vi "Remove HTML Tags from String.vi"(1 "HTML text":string) -> (0 "HTML text w/o tags":string)   [LabVIEW 2021, in "Strings.lvlib"]
uses:
  Strings/Strings.lvlib
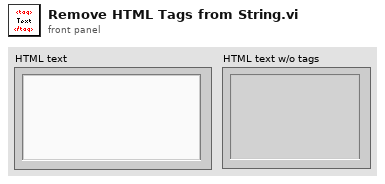
[diagram p1: front panel]
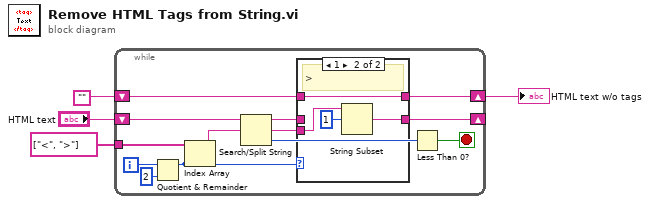
[diagram p0: block diagram]
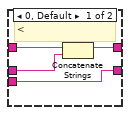
[diagram p2: hidden frame]
diagram:
  n1 = while {
    shift-right: [w7] -> _
    shift-left: "HTML text" -> [w17]
    tunnel: string[] ["<", ">"] ("search string/char (-)") -> [w14]
    shift-right: [w10] -> w1
    shift-left: "" -> [w12]
    i -> [w16]
    stop <- w5 stop-if-true
    n2 = Quotient & Remainder(x=w16, y=2) -> (x-y*floor(x/y)=w9:i32)  [unwired: 1 out]
    n3 = Index Array(array=w14, index=w9) -> (element=w13:string)
    n4 = Search/Split String(string=w17, search string/char (-)=w13) -> (substring before match=w11:string, match + rest of string=w8:string, offset of match=w6:i32)  [unwired: 1 in]
    n5 = case shown="1" w9 {
      tunnel: w12 -> [w21 w24]
      tunnel: w11 -> [w20 _]
      tunnel: [w19 w24] -> w10
      tunnel: w8 -> [w18 w25]
      tunnel: [w18 w23] -> w7
      frame 0, Default {
        # "<"
        n6 = Concatenate Strings(w21, w20) -> (w19:string)
      }
      frame 1 {
        # ">"
        n7 = String Subset(string=w25, offset (0)=1) -> (substring=w23:string)  [unwired: 1 in]
      }
    }
    n8 = Less Than 0?(x=w6) -> (x < 0?=w5:bool)
  }
  "HTML text w/o tags" <- w1
